vi "oa_Extract Waveform Segment (1 Channel).vi"(0 "scaled signal [EU]":waveform(dbl)={"t0"=timestamp(0 s since 1904-01-01), "dt"=0.0, "Y"=[]}, 1 "reset? (True)":bool=TRUE, 2 "processed time in":dbl, 5 "pulse positions [s]":dbl[](array[numeric]) format="%.2f", 7 "pulse/revolution (1)":i32=1, 11 "error in (no error)":errorcluster) -> (3 "processed time out":dbl, 4 "signal out":dbl[](array[numeric]), 6 "dt":dbl, 8 "start":i32[](array[numeric]), 10 "durations":i32[](array[numeric]), 15 "error out":errorcluster)   [LabVIEW 2017, in "SoundVib_RefDataProcess.lvlib"]
uses:
  <vilib>/addons/Sound and Vibration/Order Analysis/Referece Data Processing/SoundVib_RefDataProcess.lvlib
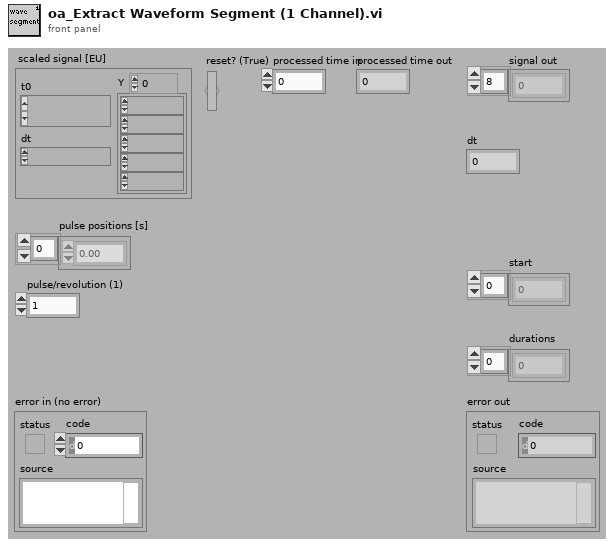
[diagram p1: front panel]
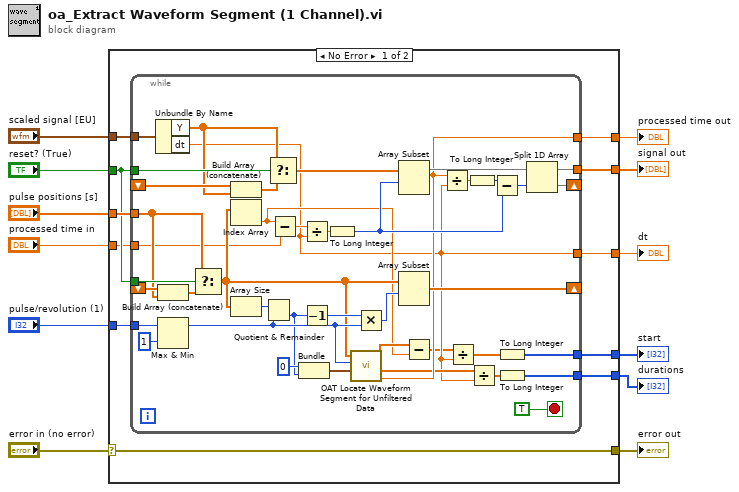
[diagram p0: block diagram]
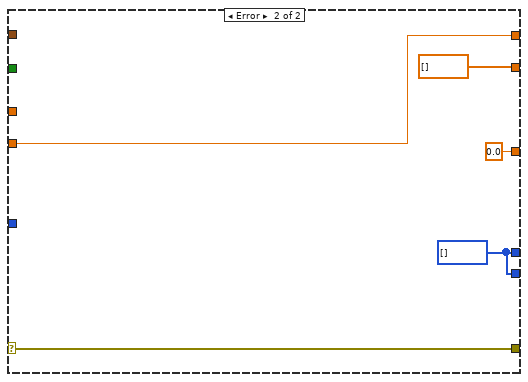
[diagram p2: hidden frame]
diagram:
  n1 = case shown="No Error" "error in (no error)" {
    selector: "error in (no error)" -> [w19 w70]
    tunnel: [w19 w70] -> w11
    tunnel: "scaled signal [EU]" -> [w18 _]
    tunnel: "reset? (True)" -> [w17 _]
    tunnel: "pulse positions [s]" -> [w22 _]
    tunnel: "pulse/revolution (1)" -> [w23 _]
    tunnel: [w21 w67] -> w6
    tunnel: [w20 w67] -> w5
    tunnel: "processed time in" -> [w16 w68]
    tunnel: [w15 dbl[] [] ("start points")] -> w3
    tunnel: [w14 w68] -> w2
    tunnel: [w13 0.0 ("dt")] -> w1
    frame No Error {
      n2 = while {
        tunnel: w23 -> [w64]
        tunnel: w22 -> [w47]
        shift-right: [w62] -> _
        shift-left: _ -> [w59]
        tunnel: [w28] -> w21
        tunnel: [w27] -> w20
        tunnel: w17 -> [w61]
        tunnel: w17 -> [w50]
        tunnel: w18 -> [w51]
        shift-right: [w38] -> _
        shift-left: _ -> [w49]
        tunnel: w16 -> [w32]
        tunnel: [w40] -> w15
        tunnel: [w34] -> w14
        tunnel: [w26] -> w13
        stop <- TRUE stop-if-true
        n3 = Unbundle By Name(w51) -> ("Y"=w46:dbl[], "dt"=w26:dbl)
        n4 = Build Array (concatenate)(w59, w47) -> (w60:dbl[])
        n5 = Max & Min(x=w64, y=1) -> (max(x,y)=w54:i32)  [unwired: 1 out]
        n6 = Select(t=w47, s=w61, f=w60) -> (s? t:f=w45:dbl[])
        n7 = Build Array (concatenate)(w49, w46) -> (w48:dbl[])
        n8 = Index Array(array=w45) -> (element=w29:dbl)  [unwired: 1 in]
        n9 = Array Size(array=w45) -> (size(s)=w55:i32)
        n10 = Quotient & Remainder(x=w55, y=w54) -> (floor(x/y)=w53:i32)  [unwired: 1 out]
        n11 = Select(t=w46, s=w50, f=w48) -> (s? t:f=w39:dbl[])
        n12 = Subtract(x=w29, y=w32) -> (x-y=w44:dbl)
        n13 = Bundle(0, w53) -> (w58:cluster{i32, i32})  [unwired: 1 in]
        n14 = Divide(x=w44, y=w26) -> (x/y=w43:dbl)
        n15 = Decrement(x=w53) -> (x-1=w52:i32)
        n16 = To Long Integer(number=w43) -> (32bit integer=w36:i32)
        n17 = call <vilib>:"OAT Locate Waveform Segment for Unfiltered Data.vi"("revolutions to display"=w58, "pulse/revolution (1)"=w54, "pulse positions [s]"=w45) -> ("last point"=w34:dbl, "durations"=w31:dbl[], "start points"=w33:dbl[])  [unwired: 5 in, 1 out]
        n18 = Multiply(x=w52, y=w54) -> (x*y=w56:i32)
        n19 = Array Subset(array=w39, index=w36) -> (w41:dbl[])  [unwired: 1 in]
        n20 = Array Subset(array=w45, index=w56) -> (w62:dbl[])  [unwired: 1 in]
        n21 = Subtract(x=w33, y=w29) -> (x-y=w25:dbl[])
        n22 = Divide(x=w34, y=w26) -> (x/y=w42:dbl)
        n23 = Divide(x=w25, y=w26) -> (x/y=w24:dbl[])
        n24 = To Long Integer(number=w42) -> (32bit integer=w37:i32)
        n25 = Divide(x=w31, y=w26) -> (x/y=w30:dbl[])
        n26 = Subtract(x=w37, y=w36) -> (x-y=w35:i32)
        n27 = To Long Integer(number=w24) -> (32bit integer=w28:i32[])
        n28 = To Long Integer(number=w30) -> (32bit integer=w27:i32[])
        n29 = Split 1D Array(array=w41, index=w35) -> (first subarray=w40:dbl[], second subarray=w38:dbl[])
      }
    }
    frame Error {
      w67 = i32[] []
    }
  }
  "error out" <- w11
  "start" <- w6
  "durations" <- w5
  "processed time out" <- w2
  "signal out" <- w3
  "dt" <- w1
